vi "convToConfigData.vi"(5 "Raw Config in":u16[](array[numeric])) -> (2 "Config out":T1)   [LabVIEW 2010, in "TPVG_DLL.lvlib"]
doc: "------------------------------------------\nAuthor: Dang Lam\nEmail: danglamtd@gmail.com"
uses:
  TPVG_DLL.lvlib
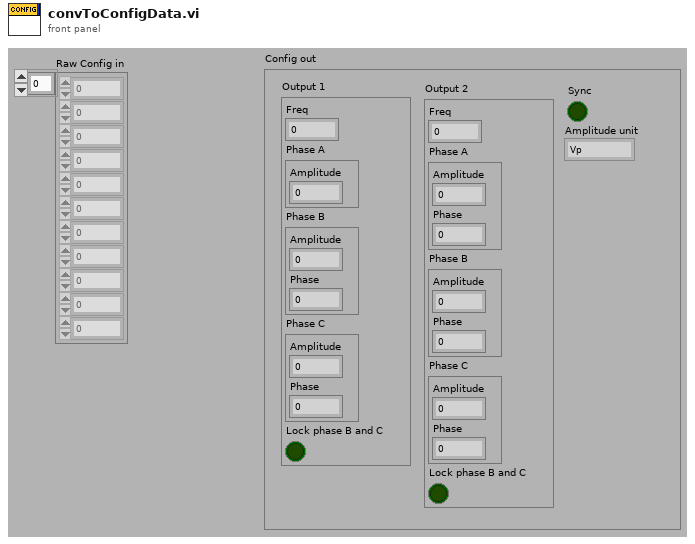
[diagram p1: front panel]
types:
  T1 = cluster{"Output 1":cluster{"Freq":sgl, "Phase A":cluster{"Amplitude":sgl}, "Phase B":cluster{"Amplitude":sgl, "Phase":sgl}, "Phase C":cluster{"Amplitude":sgl, "Phase":sgl}, "Lock":bool}, "Output 2":cluster{"Freq":sgl, "Phase A":cluster{"Amplitude":sgl, "Phase":sgl}, "Phase B":cluster{"Amplitude":sgl, "Phase":sgl}, "Phase C":cluster{"Amplitude":sgl, "Phase":sgl}, "Lock":bool}, "Sync":bool, "Amplitude unit":enum16{"Vp", "Vp-p", "Vrms"}}
  T2 = cluster{dbl, cluster{dbl}, cluster{dbl, dbl}, cluster{dbl, dbl}, bool}
  T3 = cluster{dbl, cluster{dbl, dbl}, cluster{dbl, dbl}, cluster{dbl, dbl}, bool}
  T4 = cluster{cluster{dbl, cluster{dbl}, cluster{dbl, dbl}, cluster{dbl, dbl}, bool}, cluster{dbl, cluster{dbl, dbl}, cluster{dbl, dbl}, cluster{dbl, dbl}, bool}, bool, u16}
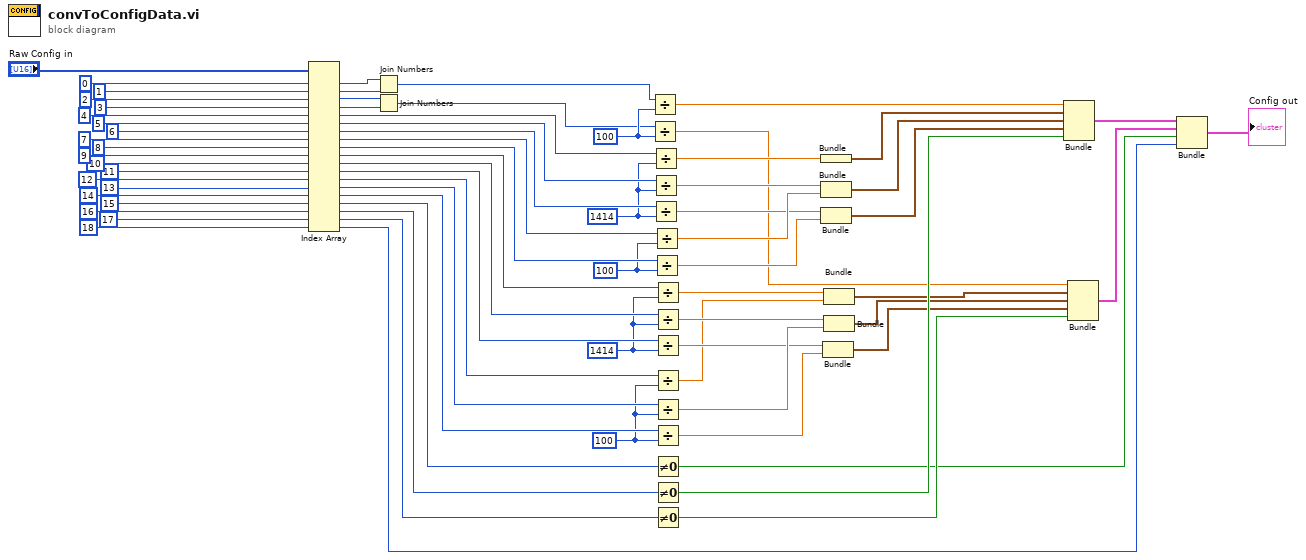
[diagram p0: block diagram]
diagram:
  w5 = u16 100 ("y")
  w51 = u16 1414 ("y")
  w58 = u16 100 ("y")
  w63 = u16 1414 ("y")
  w67 = u16 100 ("y")
  n1 = Index Array(array="Raw Config in", index #1=0 ("index"), index #2=1 ("index"), index #3=2 ("index"), index #4=3 ("index"), index #5=4 ("index"), index #6=5 ("index"), index #7=6 ("index"), index #8=7 ("index"), index #9=8 ("index"), index #10=9 ("index"), index #11=10 ("index"), index #12=11 ("index"), index #13=12 ("index"), index #14=13 ("index"), index #15=14 ("index"), index #16=15 ("index"), index #17=16 ("index"), index #18=17 ("index"), index #19=18 ("index")) -> (element #1=w23:u16, element #2=w24:u16, element #3=w18:u16, element #4=w19:u16, element #5=w66:u16, element #6=w65:u16, element #7=w64:u16, element #8=w60:u16, element #9=w59:u16, element #10=w54:u16, element #11=w53:u16, element #12=w52:u16, element #13=w3:u16, element #14=w6:u16, element #15=w7:u16, element #16=w8:u16, element #17=w9:u16, element #18=w10:u16, element #19=w1:u16)
  n2 = Join Numbers(hi=w23, lo=w24) -> ((hi.lo)=w22:u32)
  n3 = Join Numbers(hi=w18, lo=w19) -> ((hi.lo)=w17:u32)
  n4 = Divide(x=w22, y=w67) -> (x/y=w44:dbl)
  n5 = Divide(x=w17, y=w67) -> (x/y=w43:dbl)
  n6 = Divide(x=w66, y=w63) -> (x/y=w46:dbl)
  n7 = Divide(x=w65, y=w63) -> (x/y=w50:dbl)
  n8 = Divide(x=w64, y=w63) -> (x/y=w48:dbl)
  n9 = Divide(x=w60, y=w58) -> (x/y=w49:dbl)
  n10 = Divide(x=w59, y=w58) -> (x/y=w47:dbl)
  n11 = Divide(x=w54, y=w51) -> (x/y=w42:dbl)
  n12 = Divide(x=w53, y=w51) -> (x/y=w39:dbl)
  n13 = Divide(x=w52, y=w51) -> (x/y=w35:dbl)
  n14 = Divide(x=w3, y=w5) -> (x/y=w4:dbl)
  n15 = Divide(x=w6, y=w5) -> (x/y=w38:dbl)
  n16 = Divide(x=w7, y=w5) -> (x/y=w34:dbl)
  n17 = Not Equal To 0?(x=w8) -> (x != 0?=w28:bool)
  n18 = Not Equal To 0?(x=w9) -> (x != 0?=w45:bool)
  n19 = Not Equal To 0?(x=w10) -> (x != 0?=w31:bool)
  n20 = Bundle(w46) -> (w41:cluster{dbl})  [unwired: 1 in]
  n21 = Bundle(w50, w49) -> (w37:cluster{dbl, dbl})  [unwired: 1 in]
  n22 = Bundle(w48, w47) -> (w33:cluster{dbl, dbl})  [unwired: 1 in]
  n23 = Bundle(w35, w34) -> (w32:cluster{dbl, dbl})  [unwired: 1 in]
  n24 = Bundle(w42, w4) -> (w40:cluster{dbl, dbl})  [unwired: 1 in]
  n25 = Bundle(w39, w38) -> (w36:cluster{dbl, dbl})  [unwired: 1 in]
  n26 = Bundle(w44, w41, w37, w33, w45) -> (w30:T2)  [unwired: 1 in]
  n27 = Bundle(w43, w40, w36, w32, w31) -> (w29:T3)  [unwired: 1 in]
  n28 = Bundle(w30, w29, w28, w1) -> (→"Config out":T4)  [unwired: 1 in]
